vi "Read Axis Nth Frame.vi"(11 "connection ID":refnum<k5>) -> (0 "error out":errorcluster, 2 "Raw Image Data":string, 3 "connection ID out":refnum<k5>)   [LabVIEW 2017]
panel:
  in  "error in (no error)":errorcluster
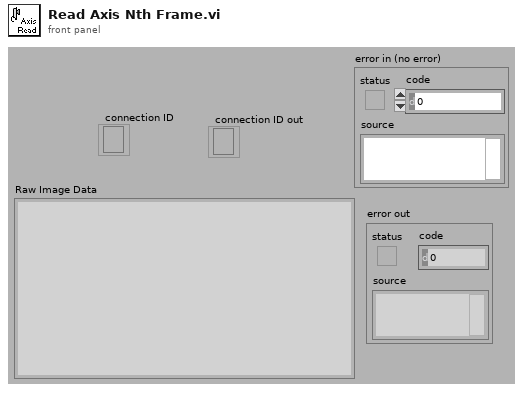
[diagram p1: front panel]
types:
  T1 = enum16{"Standard", "Buffered", "CRLF", "Immediate"}
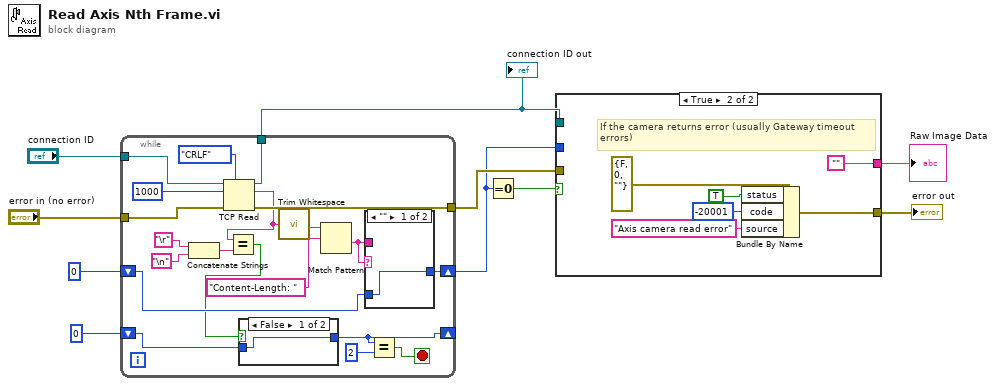
[diagram p0: block diagram]
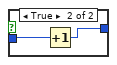
[diagram p2: hidden frame]
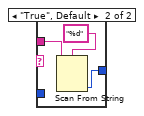
[diagram p3: hidden frame]
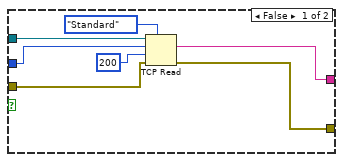
[diagram p4: hidden frame]
diagram:
  n1 = while {
    tunnel: [w28] -> w8
    tunnel: [w27] -> w7
    shift-right: [w20] -> w6
    shift-left: 0 -> [w19]
    tunnel: "connection ID" -> [w17]
    tunnel: "error in (no error)" -> [w16]
    shift-right: [w11] -> _
    shift-left: 0 -> [w12]
    stop <- w13 stop-if-true
    n2 = Concatenate Strings("\r", "\n") -> (w24:string)
    n3 = TCP Read(connection ID=w17, bytes to read=1000, error in (no error)=w16, 7:T1."CRLF" ("mode (standard)")) -> (connection ID out=w28:refnum<k5>, data out=w18:string, error out=w27:errorcluster)  [unwired: 1 in]
    n4 = Equal?(x=w18, y=w24) -> (x = y?=w15:bool)
    n5 = case shown="False" w15 {
      tunnel: w12 -> [w31 w33]
      tunnel: [w31 w32] -> w11
      frame False {
      }
      frame True {
        n6 = Increment(x=w33) -> (x+1=w32:i32)
      }
    }
    n7 = call <vilib>:"Trim Whitespace.vi"("string"=w18) -> ("trimmed string"=w22:string)  [unwired: 1 in]
    n8 = Match Pattern(string=w22, regular expression="Content-Length: ") -> (after substring=w21:string)  [unwired: 1 in, 3 out]
    n9 = case shown="\"\"" w21 {
      tunnel: w21 -> [_ w37]
      tunnel: [w34 w35] -> w20
      tunnel: w19 -> [w34 _]
      frame "" {
      }
      frame "True", Default {
        n10 = Scan From String(format string="%d", input string=w37) -> (output 1=w35:i32)  [unwired: 3 in, 3 out]
      }
    }
    n11 = Equal?(x=w11, y=2) -> (x = y?=w13:bool)
  }
  "connection ID out" <- w8
  n12 = Equal To 0?(x=w6) -> (x = 0?=w9:bool)
  n13 = case shown="True" w9 {
    tunnel: w8 -> [w44 _]
    tunnel: w7 -> [w43 _]
    tunnel: [w42 w50] -> w1
    tunnel: [w38 ""] -> w10
    tunnel: w6 -> [w39 _]
    frame False {
      n14 = TCP Read(connection ID=w44, bytes to read=w39, error in (no error)=w43, 7:T1."Standard" ("mode (standard)"), 9:200 ("timeout ms (25000)")) -> (data out=w38:string, error out=w42:errorcluster)  [unwired: 1 out]
    }
    frame True {
      # "If the camera returns error (usually Gateway timeout\nerrors)"
      n15 = Bundle By Name(cluster=errorcluster {"status"=FALSE, "code"=0, "source"=""} ("error in"), "status"=TRUE, "code"=-20001, "source"="Axis camera read error") -> (w50:errorcluster)
    }
  }
  "Raw Image Data" <- w10
  "error out" <- w1
